vi "PLC IP Address.vi"(8 "error in (no error)":errorcluster, 9 "Operationip":T2, 10 "IP Address":string, 11 "Siemens Ctr":T1) -> (0 "error out":errorcluster, 2 "Boolean":bool, 3 "Siemens Ctr out":T1)   [LabVIEW 2014, in "Simatic S7.lvlib"]
uses:
  Simatic S7.lvlib
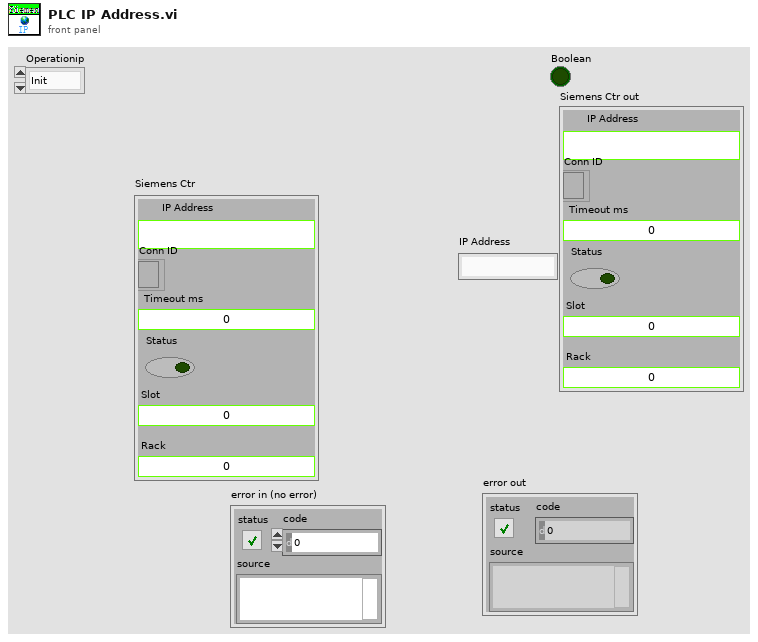
[diagram p1: front panel]
types:
  T1 = typedef "Simatic S7.lvlib/Siemens Ref.ctl" = cluster{"IP Address ":string, "Conn ID":refnum<k5>, "Timeout ms":i32, "Status":bool, "Slot":u16, "Rack":u16}
  T2 = typedef "Simatic S7.lvlib/Op ip address.ctl" = enum16{"Init", "Add IP", "Get IP"}
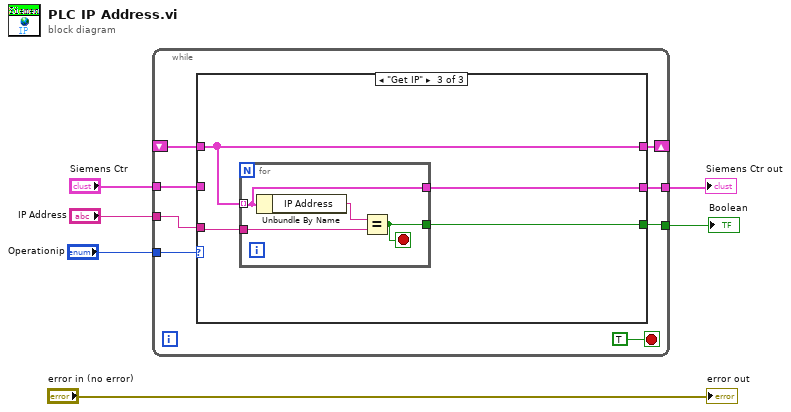
[diagram p0: block diagram]
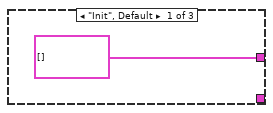
[diagram p2: hidden frame]
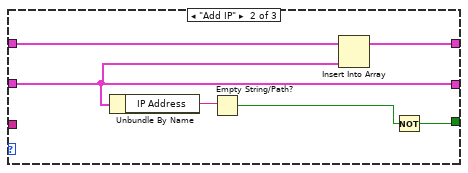
[diagram p3: hidden frame]
diagram:
  n1 = while {
    tunnel: "Operationip" -> [w13]
    shift-right: [w12] -> _
    shift-left: _ -> [w11]
    tunnel: "Siemens Ctr" -> [w10]
    tunnel: "IP Address" -> [w9]
    tunnel: [w8] -> w3
    tunnel: [w7] -> w2
    stop <- TRUE stop-if-true
    n2 = case shown="\"Get IP\"" w13 {
      tunnel: [T1[] [] w20 w25] -> w12
      tunnel: w11 -> [_ w21 w25]
      tunnel: w10 -> [_ w19 _]
      tunnel: w9 -> [_ _ w24]
      tunnel: [_ w17 w23] -> w8
      tunnel: [_ w19 w22] -> w7
      frame "Init", Default {
      }
      frame "Add IP" {
        n3 = Unbundle By Name(w19) -> ("IP Address"=w18:string)
        n4 = Empty String/Path?(string/path=w18) -> (empty?=w16:bool)
        n5 = Insert Into Array(array=w21, new element=w19) -> (w20:T1[])  [unwired: 1 in]
        n6 = Not(x=w16) -> (.not. x?=w17:bool)
      }
      frame "Get IP" {
        n7 = for {
          tunnel: w25 -> [w26] mode=indexing
          tunnel: w24 -> [w28]
          tunnel: [w27] -> w23
          tunnel: [w26] -> w22
          stop <- w27 stop-if-true
          n8 = Unbundle By Name(w26) -> ("IP Address"=w29:string)
          n9 = Equal?(x=w29, y=w28) -> (x = y?=w27:bool)
        }
      }
    }
  }
  "Boolean" <- w3
  "Siemens Ctr out" <- w2
  "error out" <- "error in (no error)"
